vi "OPCServerConnect.vi"() -> (0 "OPC UA client refnum out":T1)   [LabVIEW 2025]
uses:
  <vilib>/OPCUA/NI OPC UA Client.lvlib
  <vilib>/Utility/config.llb/NI_LVConfig.lvlib
  <vilib>/Utility/config.llb/Read Key (String).vi
  <vilib>/OPCUA/client/Connect2.vi
  <vilib>/OPCUA/controls/OPC UA Client Refnum.ctl
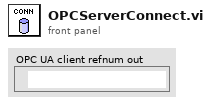
[diagram p1: front panel]
types:
  T1 = typedef "OPC UA Client Refnum.ctl" = refnum<k21>
  T2 = cluster{"message mode":enum16{"None", "Sign", "Sign and Encrypt"}, "security":enum16{"Basic256Sha256", "Aes128Sha256RsaOaep", "Aes256Sha256RsaPss"}}
  T3 = typedef "NI_LVConfig.lvlib/Config Data RefNum.ctl" = refnum<k1>
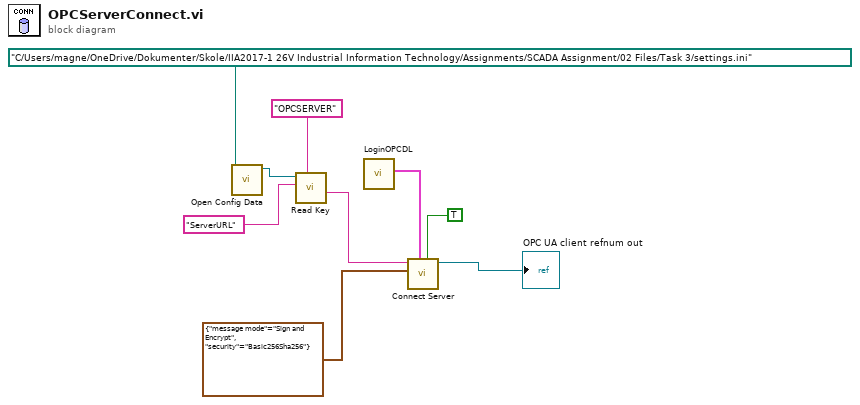
[diagram p0: block diagram]
diagram:
  n1 = call <vilib>:"Open Config Data.vi"("configuration file path"=path "C:/Users/magne/OneDrive/Dokumenter/Skole/IIA2017-1 26V Industrial Information Technology/Assignments/SCADA Assignment/02 Files/Task 3/settings.ini") -> ("refnum"=w7:T3)  [unwired: 8 in, 2 out]
  n2 = call-poly <vilib>:"Read Key.vi"("section"="OPCSERVER", "key"="ServerURL", "refnum"=w7) -> ("value"=w4:string)  [unwired: 5 in, 3 out]
  n3 = call "LoginOPCDL.vi"() -> ("output cluster"=w1:cluster{"Username":string, "Password":string})  [unwired: 11 in]
  n4 = call-poly <vilib>:"Connect Server.vi"("trust any server (F)"=TRUE, "username/password"=w1, "security policy"=T2 {"message mode"=enum."Sign and Encrypt", "security"=enum."Basic256Sha256"}, "server endpoint URL"=w4) -> ("OPC UA client refnum out"=→"OPC UA client refnum out":T1)  [unwired: 5 in, 2 out]
